vi "Do Something.vi"(8 "error in (no error)":errorcluster, 11 "ByRef Base in":refnum<class "ByRef Base.lvclass">) -> (0 "error out":errorcluster, 3 "ByRef Base out":refnum<class "ByRef Base.lvclass">)   [LabVIEW 2020, in "ByRef Base.lvclass"]
uses:
  ByRef Base.lvclass
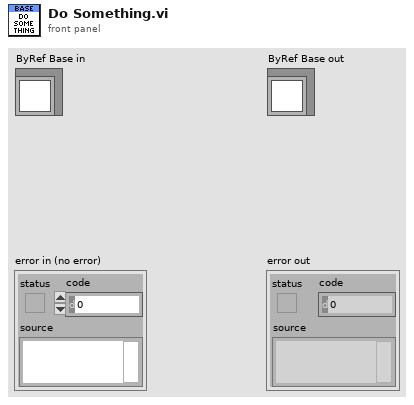
[diagram p1: front panel]
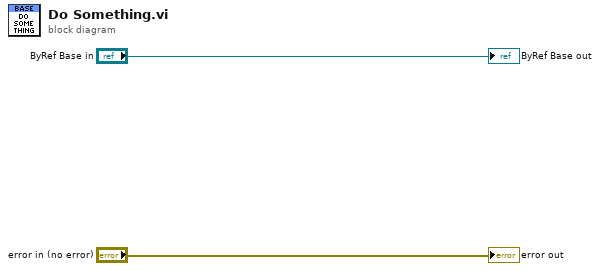
[diagram p0: block diagram]
diagram:
  "error out" <- "error in (no error)"
  "ByRef Base out" <- "ByRef Base in"
